vi "MJGPID_v2.vi"(8 "PID Gains":cluster{"Kp":dbl, "Kd":dbl, "Ki":dbl}, 10 "Encoder Position":i32, 11 "Reference":dbl) -> (2 "Direction":bool, 3 "Duty Cycle":dbl)   [LabVIEW 2016]
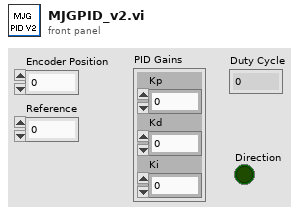
[diagram p1: front panel]
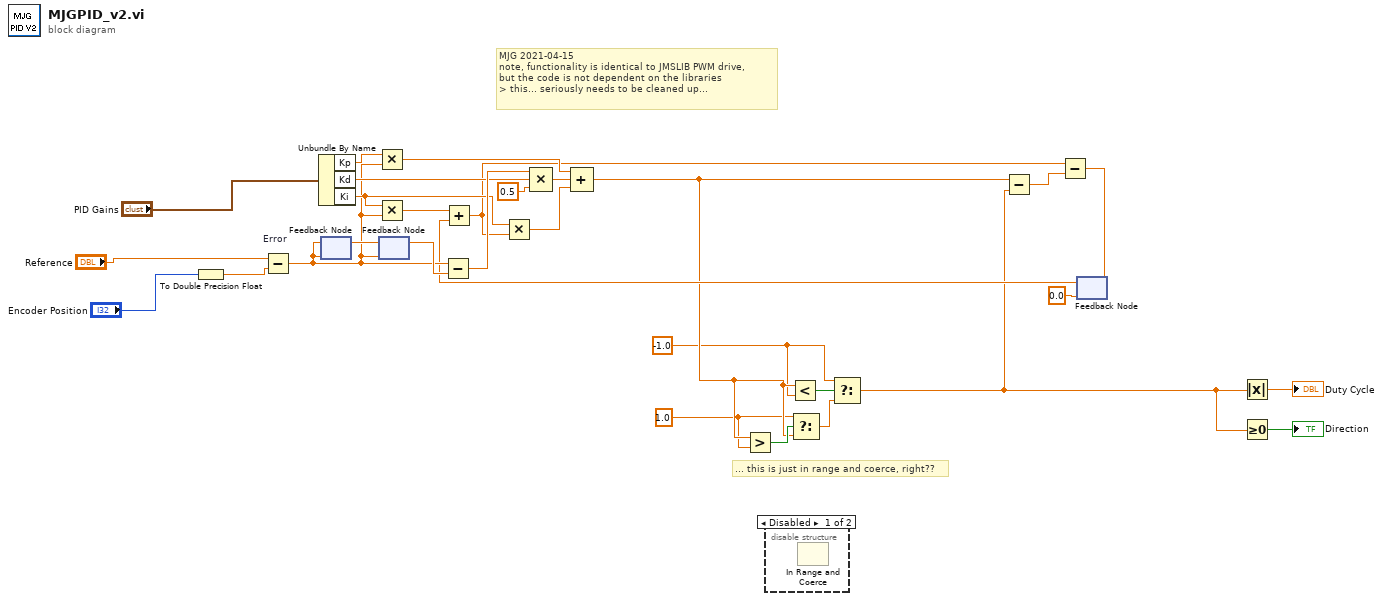
[diagram p0: block diagram]
diagram:
  w5 = 1.0 ("t")
  w6 = -1.0 ("t")
  # "... this is just in range and coerce, right??"
  # "MJG 2021-04-15\nnote, functionality is identical to JMSLIB PWM drive, \nbut the code is not dependent on the libraries\n> this... seriously needs to be cleaned up..."
  n1 = To Double Precision Float(number="Encoder Position") -> (double precision float=w4:dbl)
  n2 = Subtract "Error"(x="Reference", y=w4) -> (x-y=w18:dbl)
  n3 = Unbundle By Name("PID Gains") -> ("Kp"=w29:dbl, "Kd"=w24:dbl, "Ki"=w19:dbl)
  n4 = feedback #1(w18) -> (w27:dbl)
  n5 = feedback-in #1(w18) -> ()
  n6 = Multiply(x=w29, y=w18) -> (x*y=w28:dbl)
  n7 = Multiply(x=w19, y=w18) -> (x*y=w17:dbl)
  n8 = feedback #2(w18) -> (w26:dbl)
  n9 = feedback-in #2(w27) -> ()
  n10 = Subtract(x=w18, y=w26) -> (x-y=w25:dbl)
  n11 = Compound Arithmetic op=MULTIPLY(w25, w24, 0.5 ("value")) -> (w22:dbl)
  n12 = disable-structure shown="Disabled" {
    frame Disabled {
      n13 = In Range and Coerce() -> ()  [unwired: 3 in, 2 out]
    }
    frame Enabled {
    }
  }
  n14 = feedback #3(0.0 ("value")) -> (w16:dbl)
  n15 = Add(x=w17, y=w16) -> (x+y=w14:dbl)
  n16 = Multiply(x=w19, y=w14) -> (x*y=w20:dbl)
  n17 = Compound Arithmetic op=ADD(w28, w22, w20) -> (w7:dbl)
  n18 = Greater?(x=w7, y=w5) -> (0:w10:bool)
  n19 = Less?(x=w7, y=w6) -> (x < y?=w9:bool)
  n20 = Select(t=w5, s=w10, f=w7) -> (s? t:f=w8:dbl)
  n21 = Select(t=w6, s=w9, f=w8) -> (s? t:f=w2:dbl)
  n22 = Subtract(x=w7, y=w2) -> (x-y=w15:dbl)
  n23 = Subtract(x=w14, y=w15) -> (x-y=w13:dbl)
  n24 = feedback-in #3(w13) -> ()
  n25 = Absolute Value(x=w2) -> (abs(x)=→"Duty Cycle":dbl)
  n26 = Greater Or Equal To 0?(x=w2) -> (x >= 0?=→"Direction":bool)
